vi "Get Path.vi"(8 "error in (no error)":errorcluster, 9 "channel 2":string, 10 "channel 1":string, 11 "session in":T1) -> (0 "error out":errorcluster, 2 "path":string, 3 "session out":T1)   [LabVIEW 2020, in "SLSC Switch.lvlib"]
doc: "Returns a string that identifies the explicit path created with SLSC Switch.lvlib:Connect Channels. Pass this string to SLSC Switch.lvlib:Set Path to establish the exact same path in future connections."
uses:
  <vilib>/SLSC_Switch/SLSC Switch.lvlib
  nislscsl.dll
  <vilib>/userdefined/High Color/SLSC_Switch/nislscslSession.ctl
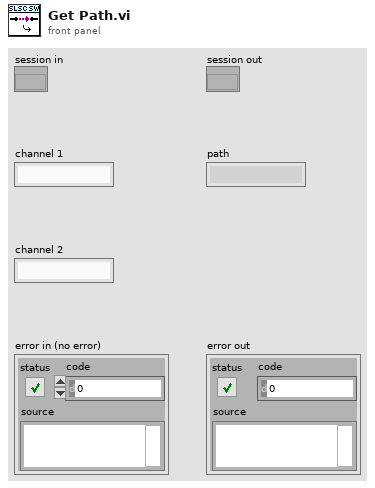
[diagram p1: front panel]
types:
  T1 = typedef "nislscslSession.ctl" = refnum<k20>
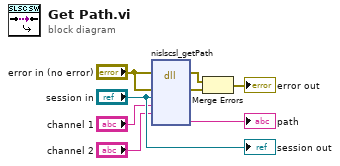
[diagram p0: block diagram]
diagram:
  n1 = dll-call lib="nislscsl.*" fn="nislscsl_getPath"(error in="error in (no error)", "errorCluster"="error in (no error)", "sessionHandle"="session in", "channel 1"="channel 1", "channel 2"="channel 2") -> (error out=w8:errorcluster, "errorCluster"=w7:errorcluster, "path"=→"path":string)  [unwired: 7 in, 1 out]
  n2 = Merge Errors(w8, w7) -> (→"error out":errorcluster)
  "session out" <- "session in"
